vi "elinqueue.vi"() -> ()   [LabVIEW 2010]
panel:
  out "# elements in queue":i32
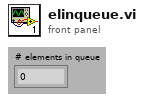
[diagram p1: front panel]
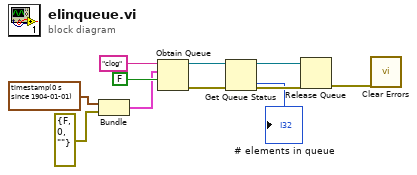
[diagram p0: block diagram]
diagram:
  n1 = Bundle(timestamp(0 s since 1904-01-01), "error out"=errorcluster {"status"=FALSE, "code"=0, "source"=""}) -> (w1:cluster{timestamp, "error out":errorcluster})  [unwired: 1 in]
  n2 = Obtain Queue(name (unnamed)="clog", element data type=w1, create if not found? (T)=FALSE) -> (queue out=w9:refnum<queue>, error out=w11:errorcluster)  [unwired: 2 in, 1 out]
  n3 = Get Queue Status(queue=w9, error in (no error)=w11) -> (queue out=w8:refnum<queue>, error out=w10:errorcluster, # elements in queue=→"# elements in queue":i32)  [unwired: 1 in, 5 out]
  n4 = Release Queue(queue=w8, error in (no error)=w10) -> (error out=w5:errorcluster)  [unwired: 1 in, 2 out]
  n5 = call <vilib>:"Clear Errors.vi"("error in (no error)"=w5) -> ()  [unwired: 6 in, 1 out]
